vi "SetVisibillitySettings.vi"(0 "reference":refnum<class "ClassNode.lvclass">, 1 "showAttribute":bool, 2 "showMethods":bool, 5 "error in (no error)":errorcluster) -> (14 "reference out":refnum<class "ClassNode.lvclass">, 19 "error out":errorcluster)   [LabVIEW 2014, in "ClassNode.lvclass"]
doc: "SetVisibillitySettings"
uses:
  <resource>/Framework/Providers/Open_GDS/UML/ClassNode_class/ClassNode.lvclass
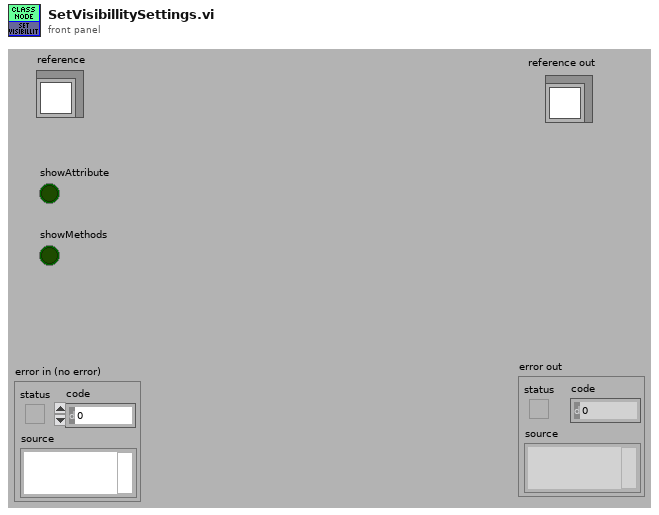
[diagram p1: front panel]
types:
  T1 = typedef "ClassNode.lvclass/ObjectAttributes.ctl" = cluster{"Base class":T2, "midHeight":dbl, "botHeight":dbl, "name":refnum<class "MultiLineString.lvclass">, "attributes":refnum<class "MultiLineString.lvclass">, "methods":refnum<class "MultiLineString.lvclass">, "DEFAULT_COMPARTMENT_HEIGHT":i32, "DEFAULT_WIDTH":i32, "DEFAULT_HEIGHT":i32, "showMethods":bool, "showAttributes":bool, "ClassPath":path}
  T2 = typedef "RectangularNode.lvclass/ObjectAttributes.ctl" = cluster{"Base class":T3, "bounds":T4}
  T3 = typedef "AbstractNode.lvclass/ObjectAttributes.ctl" = cluster{"parent":refnum<class "AbstractNode.lvclass">, "children":refnum<class "AbstractNode.lvclass">[], "Hidden":bool}
  T4 = typedef "Rectangle Rectangle2D.ctl" = cluster{"x":dbl, "y":dbl, "width":dbl, "height":dbl}
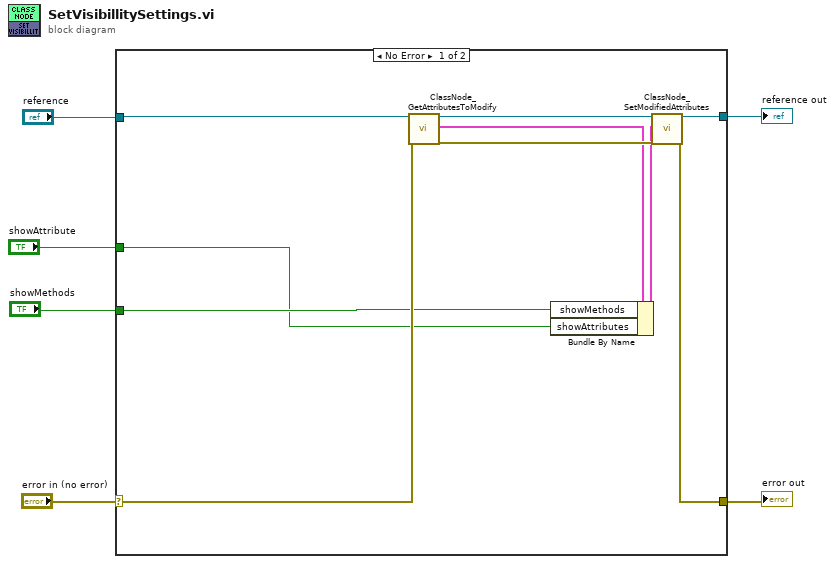
[diagram p0: block diagram]
diagram:
  n1 = case shown="No Error" "error in (no error)" {
    selector: "error in (no error)" -> [w16 w17]
    tunnel: "reference" -> [w15 w18]
    tunnel: [w10 w17] -> w4
    tunnel: [w9 w18] -> w3
    tunnel: "showMethods" -> [w8 _]
    tunnel: "showAttribute" -> [w7 _]
    frame No Error {
      n2 = call <resource>:"ClassNode_GetAttributesToModify.vi"("reference in"=w15, "error in (no error)"=w16) -> ("reference out"=w13:refnum<class "ClassNode.lvclass">, "Attributes"=w12:T1, "error out"=w14:errorcluster)  [unwired: 1 in, 14 out]
      n3 = Bundle By Name(cluster=w12, "showMethods"=w8, "showAttributes"=w7) -> (w11:T1)
      n4 = call <resource>:"ClassNode_SetModifiedAttributes.vi"("reference in"=w13, "Attributes"=w11, "error in (no error)"=w14) -> ("reference out"=w9:refnum<class "ClassNode.lvclass">, "error out"=w10:errorcluster)  [unwired: 3 in, 12 out]
    }
    frame Error {
    }
  }
  "reference out" <- w3
  "error out" <- w4
